vi "Plugin_SpecPage.vi"(10 "Spec Page Interface":T5, 11 "MetaDataObj in":refnum<class "MetaDataObj.lvclass">) -> (3 "MetaDataObj out":refnum<class "MetaDataObj.lvclass">)   [LabVIEW 2021, in "Plugin_Generator.lvclass"]
uses:
  Plugin_Generator.lvclass
  <resource>/dialog/NewProjectWizard/Spec Page Interface.ctl
  <resource>/dialog/NewProjectWizard/MetaDataObj/MetaDataObj.lvclass
  <vilib>/CIF Foundation/CIF LabVIEW Scripting/LV Scripting/Typedef/Icon Overlay.ctl
  C:/Program Files/National Instruments/LabVIEW 2021/resource/dialog/NewProjectWizard/MetaDataObj/MetaDataObj.lvclass
  <resource>/dialog/NewProjectWizard/MetaDataObj/MetaDataObj.lvclass/MetaDataObj.ctl
  Plugin_Generator.lvclass/Plugin_Generator.ctl
  <resource>/dialog/NewProjectWizard/MetaDataObj/Accessors/Write Overlay Pixmap.vi
  <resource>/dialog/NewProjectWizard/MetaDataObj/Accessors/Read Overlay Pixmap.vi
  <resource>/dialog/NewProjectWizard/MetaDataObj/Accessors/Write File Prefix.vi
  <resource>/dialog/NewProjectWizard/MetaDataObj/Accessors/Write Project Name.vi
  <resource>/dialog/NewProjectWizard/MetaDataObj/Accessors/Write Project Root.vi
  <resource>/dialog/NewProjectWizard/MetaDataObj/Accessors/Read Hide Prefix.vi
  <resource>/dialog/NewProjectWizard/MetaDataObj/Accessors/Read Hide Icon Overlay.vi
  <vilib>/LabVIEW Icon API/lv_icon/Classes/Icon/Icon.lvclass
  <vilib>/CIF Foundation/CIF LabVIEW Scripting/LV Scripting/LV Scripting Utilities.lvlib
  D:/dev/CIF-LVCore/src/CIFUtilities/Scripting/Plugin Generator/Plugin_Generator.lvclass
  <vilib>/CIF Foundation/CIF Channels Core/CIFChannels/Typedef/Direction.ctl
  <vilib>/CIF Foundation/CIF Channels Core/CIFChannels/CIFChannels.lvclass
  Channels/ChannelRegistrar/typedef/Registered Channel Types.ctl
  Channels/ChannelRegistrar/ChannelRegistrar.lvlib
  Channels/ChannelRegistrar/typedef/Channel Definition for Scripting.ctl
panel:
  in  "Channels to Create":T1[](array[typedef])
  in  "Plugin Name":string
  in  "Root Directory":path
  out "Icon":picture
  in  "Icon Customization":T4={"Text"="Plugin", "Background color"=7208704, "Text color"=0}
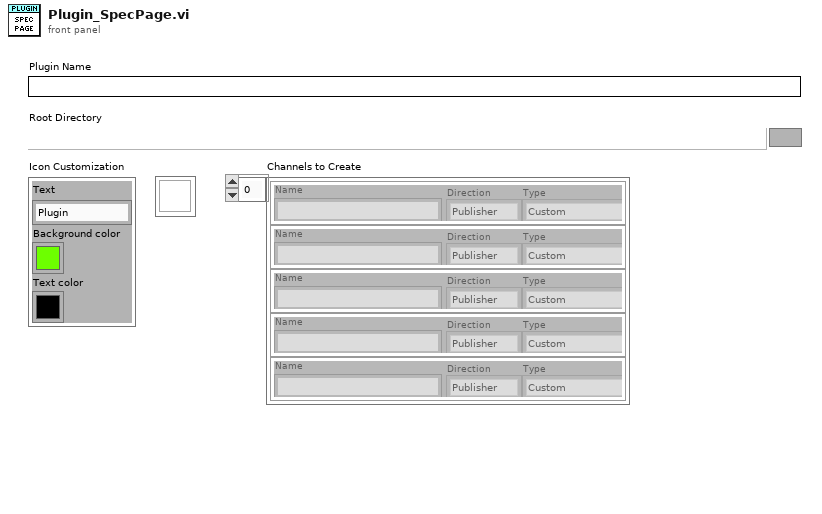
[diagram p1: front panel]
types:
  T1 = typedef "ChannelRegistrar.lvlib/Channel Definition for Scripting.ctl" = cluster{"Name":string, "Direction":T2, "Type":T3}
  T2 = typedef "CIFChannels.lvclass/Direction.ctl" = enum16{"Publisher", "Subscriber"}
  T3 = typedef "ChannelRegistrar.lvlib/Registered Channel Types.ctl" = enum16{"Custom", "Double_Tag", "I64_Tag", "U64_Tag", "U8_FIFO", "CAN_FIFO", "L2Enet_FIFO", "DAQ_FIFO", "Universal_FIFO", "String_Tag"}
  T4 = typedef "LV Scripting Utilities.lvlib/Icon Overlay.ctl" = cluster{"Text":string, "Background color":u32, "Text color":u32}
  T5 = typedef "Spec Page Interface.ctl" = cluster{"\"Tab Forward To\" Refnum":refnum<vi>, "\"Tab Backward To\" Refnum":refnum<vi>, "Errors":refnum<user-event>, "Quit":refnum<user-event>}
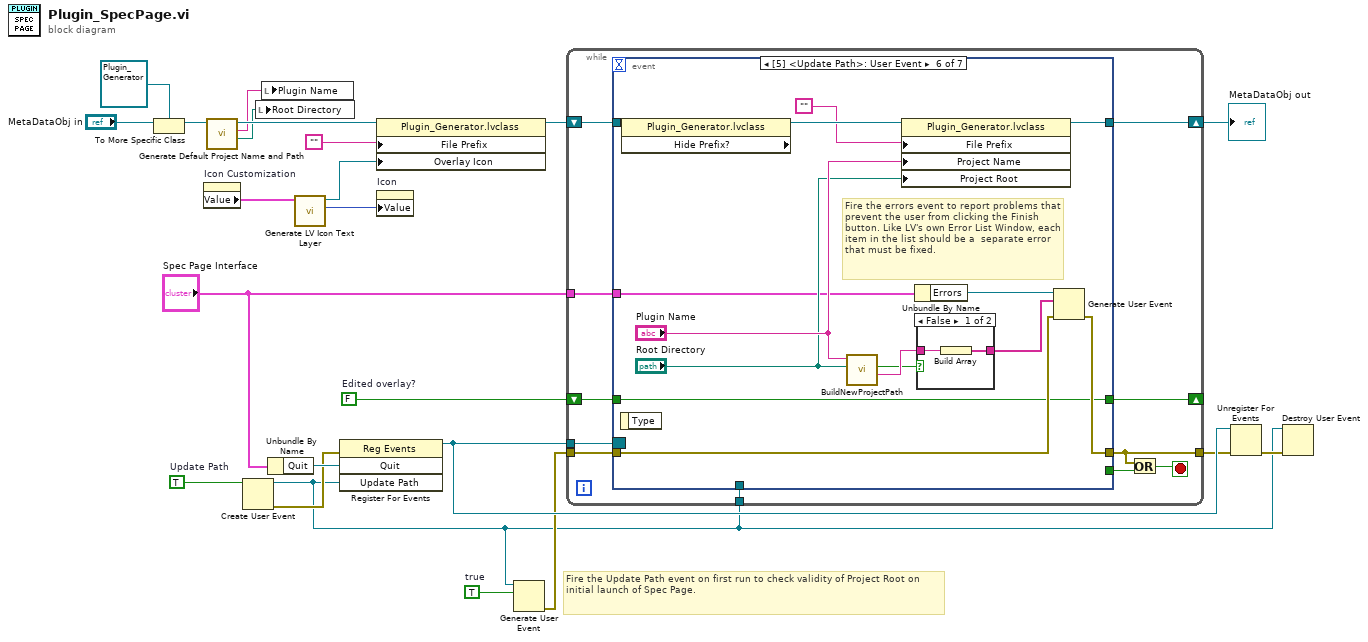
[diagram p0: block diagram]
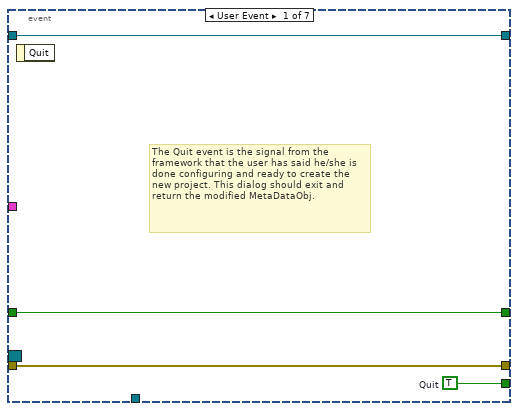
[diagram p2: hidden frame]
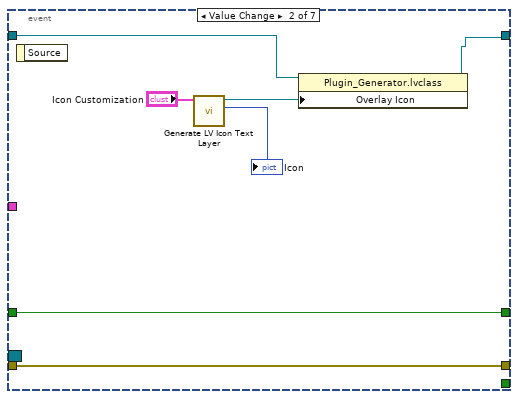
[diagram p3: hidden frame]
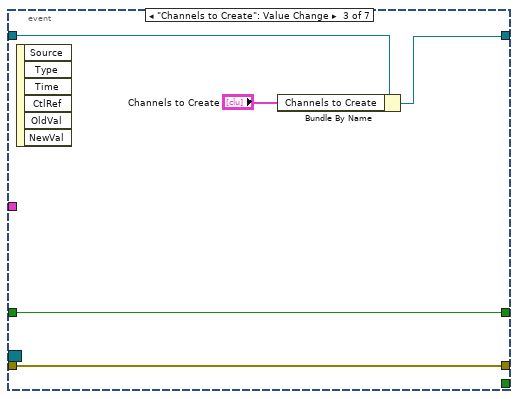
[diagram p4: hidden frame]
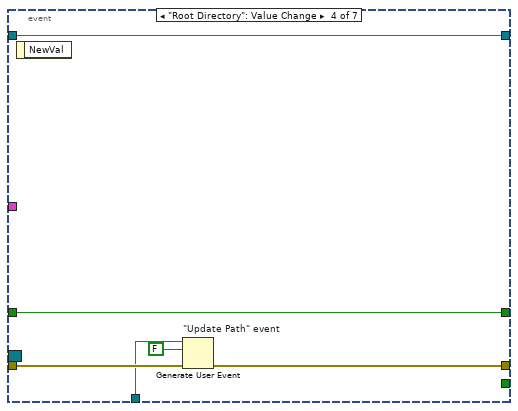
[diagram p5: hidden frame]
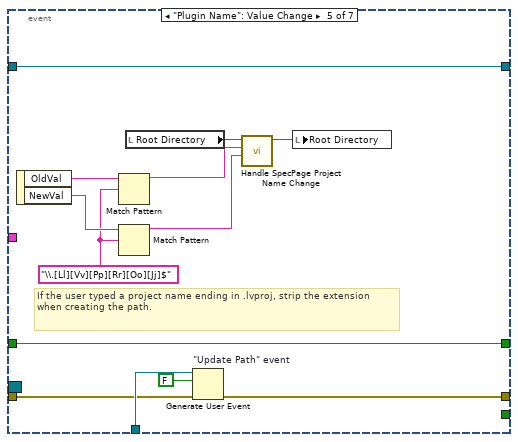
[diagram p6: hidden frame]
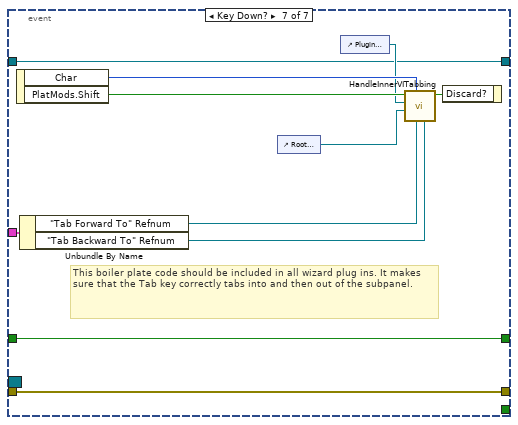
[diagram p8: hidden frame]
diagram:
  w1 = TRUE  # true
  w15 = FALSE  # Edited overlay?
  w19 = TRUE  # Update Path
  # "Fire the Update Path event on first run to check validity of Project Root on initial launch of Spec Page."
  n1 = To More Specific Class(target class=refnum<class "Plugin_Generator.lvclass"> refnum ("Plugin_Generator.lvclass"), reference="MetaDataObj in") -> (specific class reference=w4:refnum<class "Plugin_Generator.lvclass">)  [unwired: 1 in, 1 out]
  n2 = property on="Icon Customization" class="Clust (strict)"() -> ("Value"=w9:T4)  [unwired: 2 in, 2 out]
  n3 = call <resource>:"Generate Default Project Name and Path.vi"("DNL_MetaDataObj in"=w4) -> ("Project Root"=w11:path, "Project Name"=w2:string, "DNL_MetaDataObj out"=w12:refnum<class "Plugin_Generator.lvclass">)  [unwired: 8 in]
  n4 = Create User Event(user event datatype=w19) -> (user event=w13:refnum<user-event>, error out=w18:errorcluster)  [unwired: 1 in]
  n5 = local write "Root Directory"(w11) -> ()
  n6 = local write "Plugin Name"(w2) -> ()
  n7 = Unbundle By Name("Spec Page Interface") -> ("Quit"=w23:refnum<user-event>)
  n8 = call <vilib>:"Generate LV Icon Text Layer.vi"("Icon Overlay"=w9) -> ("Picture"=w8:picture, "Icon.lvlclass out"=w7:refnum<class "Icon.lvclass">)  [unwired: 8 in, 1 out]
  n9 = register-events(error in=w18, w23, w13) -> (reference out=w22:refnum<event-registration>)  [unwired: 1 in, 1 out]
  n10 = property class="Plugin_Generator.lvclass"(reference=w12, "File Prefix"="", "Overlay Icon"=w7) -> (reference out=w3:refnum<class "Plugin_Generator.lvclass">)  [unwired: 1 in, 1 out]
  n11 = property on="Icon" class="Pict"("Value"=w8) -> ()  [unwired: 2 in, 2 out]
  n12 = Generate User Event ("\"Update Path\" event")(user event=w13, event data cluster=w1) -> (error out=w14:errorcluster)  [unwired: 2 in, 1 out]
  n13 = while {
    tunnel: "Spec Page Interface" -> [w32]
    shift-right: [w31] -> w16
    shift-left: w3 -> [w30]
    tunnel: w22 -> [w34]
    tunnel: w14 -> [w33]
    tunnel: [w27] -> w20
    tunnel: w13 -> [w26]
    shift-right: [w24] -> _
    shift-left: w15 -> [w25]
    stop <- w29 stop-if-true
    n14 = event shown="[5] <Update Path>: User Event" {
      selector: w34 -> [_ _ _ _ _ _ _]
      dyn-events: _ -> [_ _ _ _ _ _ _]
      timeout: _ -> [_ _ _ _ _ _ _]
      tunnel: w32 -> [_ _ _ _ _ w77 w92]
      tunnel: [w38 _ _ _ _ _ _] -> w28
      tunnel: [w37 w45 w50 w54 w65 w75 w89] -> w27
      tunnel: w33 -> [w37 w45 w50 w55 w66 w76 w89]
      tunnel: [w36 w41 w47 w56 w62 w73 w88] -> w31
      tunnel: w30 -> [w36 w42 w48 w56 w62 w74 w88]
      tunnel: w26 -> [_ _ _ w53 w67 _ _]
      tunnel: w25 -> [w35 w44 w49 w51 w63 w72 w87]
      tunnel: [w35 w44 w49 w51 w63 w72 w87] -> w24
      event User Event {
        w38 = TRUE  # Quit
        # "The Quit event is the signal from the framework that the user has said he/she is done configuring and ready to create the new project. This dialog should exit and return the modified MetaDataObj."
        n15 = event-data() -> ()  [unwired: 1 in, 1 out]
      }
      event Value Change {
        n16 = event-data() -> ()  [unwired: 1 in, 1 out]
        n17 = call <vilib>:"Generate LV Icon Text Layer.vi"("Icon Overlay"="Icon Customization") -> ("Picture"=→"Icon":picture, "Icon.lvlclass out"=w43:refnum<class "Icon.lvclass">)  [unwired: 8 in, 1 out]
        n18 = property class="Plugin_Generator.lvclass"(reference=w42, "Overlay Icon"=w43) -> (reference out=w41:refnum<class "Plugin_Generator.lvclass">)  [unwired: 1 in, 1 out]
      }
      event "Channels to Create": Value Change {
        n19 = event-data() -> ()  [unwired: 1 in, 6 out]
        n20 = Bundle By Name(cluster=w48, "Channels to Create"="Channels to Create") -> (w47:refnum<class "Plugin_Generator.lvclass">)
      }
      event "Root Directory": Value Change {
        n21 = event-data() -> ()  [unwired: 1 in, 1 out]
        n22 = Generate User Event "\"Update Path\" event"(user event=w53, event data cluster=FALSE ("event data"), error in=w55) -> (error out=w54:errorcluster)  [unwired: 1 in, 1 out]
      }
      event "Plugin Name": Value Change {
        w57 = "\\.[Ll][Vv][Pp][Rr][Oo][Jj]$" ("regular expression")
        # "If the user typed a project name ending in .lvproj, strip the extension when creating the path."
        n23 = event-data() -> ("OldVal"=w59:string, "NewVal"=w61:string)  [unwired: 1 in]
        n24 = Match Pattern(string=w59, regular expression=w57) -> (before substring=w58:string)  [unwired: 1 in, 3 out]
        n25 = Match Pattern(string=w61, regular expression=w57) -> (before substring=w60:string)  [unwired: 1 in, 3 out]
        n26 = local read "Root Directory"() -> (w69:path)
        n27 = Generate User Event "\"Update Path\" event"(user event=w67, event data cluster=FALSE ("event data"), error in=w66) -> (error out=w65:errorcluster)  [unwired: 1 in, 1 out]
        n28 = call <resource>:"Handle SpecPage Project Name Change.vi"("Project Name New Value"=w60, "Project Name Old Value"=w58, "Project Root in"=w69) -> ("Project Root out"=w68:path)  [unwired: 8 in]
        n29 = local write "Root Directory"(w68) -> ()
      }
      event User Event {
        # "Fire the errors event to report problems that prevent the user from clicking the Finish button. Like LV's own Error List Window, each item in the list should be a  separate error that must be fixed."
        n30 = event-data() -> ()  [unwired: 1 in, 1 out]
        n31 = property class="Plugin_Generator.lvclass" props=["Hide Prefix?"](reference=w74) -> (reference out=w71:refnum<class "Plugin_Generator.lvclass">)  [unwired: 1 in, 2 out]
        n32 = call <resource>:"BuildNewProjectPath.vi"("Project Root"="Root Directory", "Project Name"="Plugin Name") -> ("Error Message"=w80:string, "Valid?"=w78:bool)  [unwired: 7 in, 1 out]
        n33 = property class="Plugin_Generator.lvclass"(reference=w71, "File Prefix"="", "Project Name"="Plugin Name", "Project Root"="Root Directory") -> (reference out=w73:refnum<class "Plugin_Generator.lvclass">)  [unwired: 1 in, 1 out]
        n34 = Unbundle By Name(w77) -> ("Errors"=w83:refnum<user-event>)
        n35 = case shown="False" w78 {
          tunnel: w80 -> [w85 _]
          tunnel: [w84 _] -> w79
          frame False {
            n36 = Build Array(w85) -> (w84:string[])
          }
          frame True {
          }
        }
        n37 = Generate User Event(user event=w83, event data cluster=w79, error in=w76) -> (error out=w75:errorcluster)  [unwired: 1 in, 1 out]
      }
      event Key Down? {
        # "This boiler plate code should be included in all wizard plug ins. It makes sure that the Tab key correctly tabs into and then out of the subpanel."
        n38 = event-data() -> ("Char"=w95:i16, "PlatMods.Shift"=w94:bool)  [unwired: 1 in]
        n39 = Unbundle By Name(w92) -> ("\"Tab Forward To\" Refnum"=w91:refnum<vi>, "\"Tab Backward To\" Refnum"=w90:refnum<vi>)
        n40 = control-ref of="Root Directory"() -> (w86:refnum<vi>)
        n41 = control-ref of="Plugin Name"() -> (w93:refnum<vi>)
        n42 = call <resource>:"HandleInnerVITabbing.vi"("Tab Backward To"=w90, "Tab Forward To"=w91, "Char"=w95, "Last Control"=w86, "First Control"=w93, "Shift"=w94) -> ("Discard"=w96:bool)  [unwired: 5 in]
        n43 = event-data("Discard?"=w96) -> ()  [unwired: 1 in, 1 out]
      }
    }
    n44 = Or(x=w27, y=w28) -> (x .or. y?=w29:bool)
  }
  "MetaDataObj out" <- w16
  n45 = Unregister For Events(event registration refnum=w22, error in=w20) -> (error out=w17:errorcluster)
  n46 = Destroy User Event(user event=w13, error in=w17) -> ()  [unwired: 1 out]
